vi "Tool Transformation.vi"(2 "SetTRF":sgl[](array[numeric])=[80.67, 0.8359, 79.37, 0.0, 0.0, 0.0] step=1 format="%.3f", 3 "External force":T1 {"£nez" format="%.3f"; "£ney" format="%.3f"; "£nex" format="%.3f"; "Fez" format="%.2f"; "Fey" format="%.2f"; "Fex" format="%.2f"}) -> (0 "Rotation Matrix":dbl[][](array[numeric]), 1 "External force":T1 {"£nez" format="%.3f"; "£ney" format="%.3f"; "£nex" format="%.3f"; "Fez" format="%.2f"; "Fey" format="%.2f"; "Fex" format="%.2f"})   [LabVIEW 2018]
uses:
  <vilib>/Analysis/coordinate.llb/Euler Rotation Order.ctl
  <vilib>/Analysis/Matrix/Datatypes/RealMatrix.ctl
  <vilib>/Analysis/baseanly.llb/A x Vector.vi
  <vilib>/Analysis/baseanly.llb/Real A x B.vi
  <vilib>/Analysis/7linalg.llb/Create Special Real Matrix.vi
  <vilib>/Analysis/NI_AALPro.lvlib
  <vilib>/Analysis/Matrix/NI_Matrix.lvlib
  <vilib>/Analysis/NI_AALBase.lvlib
panel:
  out "Force Check":dbl[](array[numeric])
  out "Torque Check":dbl[](array[numeric])
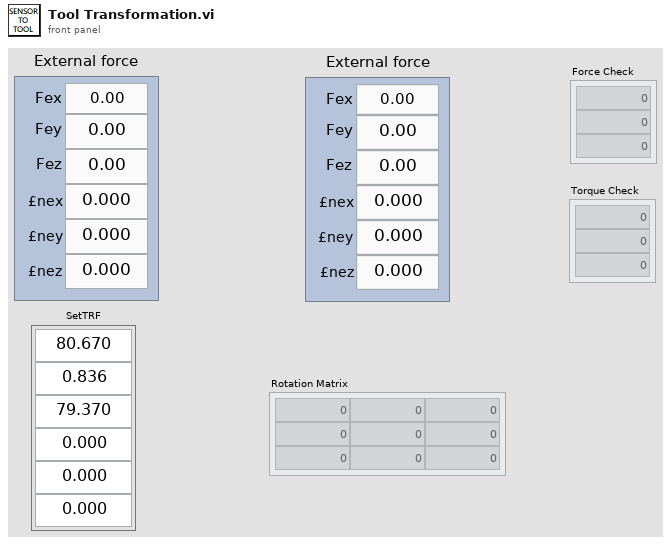
[diagram p1: front panel]
types:
  T1 = cluster{"Fex":dbl, "Fey":dbl, "Fez":dbl, " £nex":dbl, " £ney":dbl, " £nez":dbl}
  T2 = typedef "NI_Matrix.lvlib/RealMatrix.ctl" = dbl[][]
  T3 = typedef "NI_AALPro.lvlib/Euler Rotation Order.ctl" = u16
  T4 = cluster{"Move-SubIndex 1 ":sgl, "Move-SubIndex 1 ":sgl, sgl}
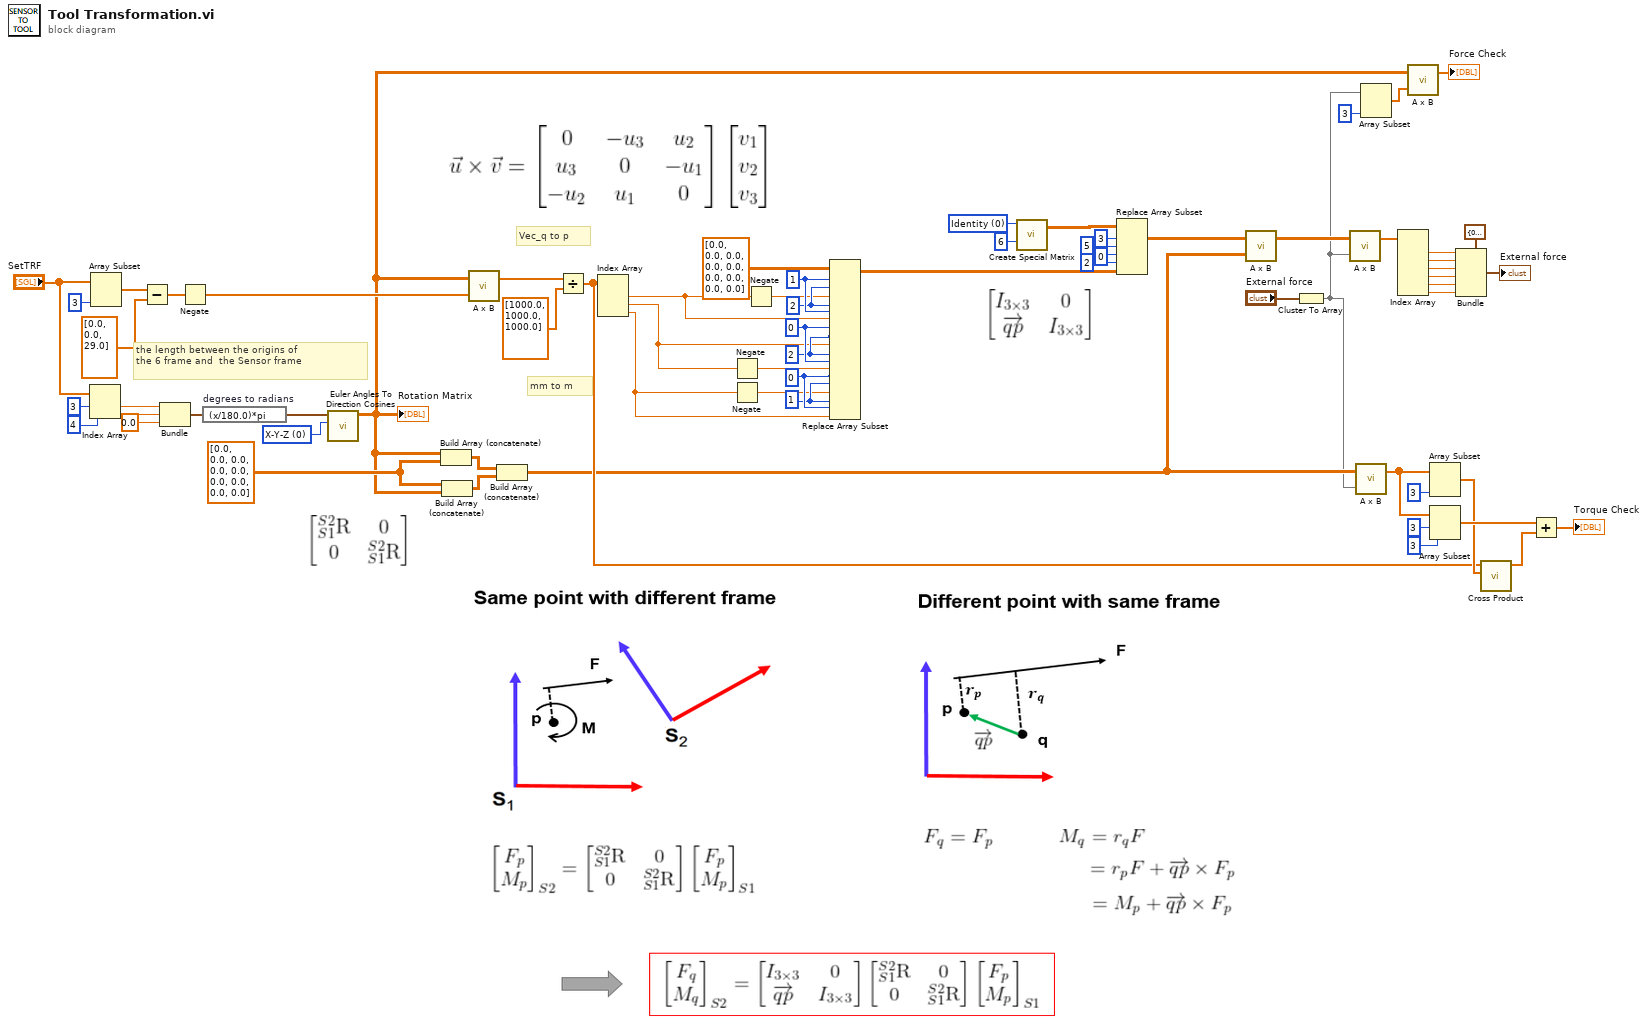
[diagram p0: block diagram]
diagram:
  w40 = T2 [[0.0, 0.0, 0.0], [0.0, 0.0, 0.0], [0.0, 0.0, 0.0]] ("matrix")
  w49 = 1 ("disabled index (col)")
  w50 = 0 ("disabled index (row)")
  w51 = 2 ("disabled index (col)")
  w52 = 0 ("disabled index (row)")
  w53 = 2 ("disabled index (col)")
  w54 = 1 ("disabled index (row)")
  w57 = 0 items=["Identity", "Diagonal", "Toeplitz", "Vandermonde", "Companion", "Hankel", "Hadamard", "Wilkinson", "Hilbert", "Inverse Hilbert", "Rosser", "Pascal"] ("matrix type")
  w66 = T3 0 items=["X-Y-Z", "X-Z-Y", "Y-X-Z", "Y-Z-X", "Z-X-Y", "Z-Y-X", "X-Y-X", "X-Z-X", "Y-X-Y", "Y-Z-Y", "Z-X-Z", "Z-Y-Z"] ("rotation order")
  # "mm to m"
  # "Vec_q to p"
  # "the length between the origins of \nthe 6 frame and  the Sensor frame"
  n1 = Index Array(array="SetTRF", index #1=3 ("index"), index #2=4 ("index")) -> (element #1=w59:sgl, element #2=w58:sgl)
  n2 = Array Subset(array="SetTRF", length=3) -> (w64:sgl[])  [unwired: 1 in]
  n3 = Subtract(x=w64, y=sgl[] [0.0, 0.0, 29.0]) -> (x-y=w12:sgl[])
  n4 = Bundle("Move-SubIndex 1"=w59, "Move-SubIndex 1"=w58, sgl 0.0) -> (w29:T4)  [unwired: 1 in]
  n5 = Negate(x=w12) -> (-x=w9:sgl[])
  n6 = expression code="(x/180.0)*pi" "degrees to radians"(w29) -> (w28:T4)
  n7 = call <vilib>:"Euler Angles To Direction Cosines.vi"("rotation order"=w66, "Euler Angles"=w28) -> ("Direction Cosines"=w1:dbl[][])  [unwired: 8 in, 1 out]
  "Rotation Matrix" <- w1
  n8 = Build Array (concatenate)(w1, w40) -> (w42:T2)
  n9 = Build Array (concatenate)(w40, w1) -> (w41:T2)
  n10 = call-poly <vilib>:"A x B.vi"("Vector"=w9, "A"=w1) -> ("A x Vector"=w8:dbl[])  [unwired: 1 out]
  n11 = Build Array (concatenate)(w42, w41) -> (w7:T2)
  n12 = Divide(x=w8, y=sgl[] [1000.0, 1000.0, 1000.0]) -> (x/y=w11:dbl[])
  n13 = Index Array(array=w11) -> (element #1=w25:dbl, element #2=w26:dbl, element #3=w22:dbl)  [unwired: 3 in]
  n14 = Negate(x=w26) -> (-x=w24:dbl)
  n15 = Negate(x=w22) -> (-x=w23:dbl)
  n16 = Negate(x=w25) -> (-x=w27:dbl)
  n17 = Replace Array Subset(array=T2 [[0.0, 0.0, 0.0], [0.0, 0.0, 0.0], [0.0, 0.0, 0.0]] ("matrix"), new element #1=w27, index (row) #1=w54, index (col) #1=w53, new element #2=w25, index (row) #2=w53, index (col) #2=w54, new element #3=w26, index (row) #3=w52, index (col) #3=w51, new element #4=w24, index (row) #4=w51, index (col) #4=w52, new element #5=w23, index (row) #5=w50, index (col) #5=w49, new element #6=w22, index (row) #6=w49, index (col) #6=w50) -> (w48:T2)
  n18 = call-poly <vilib>:"Create Special Matrix.vi"("matrix type"=w57, "matrix size"=6) -> ("Special Matrix"=w55:T2)  [unwired: 3 in, 1 out]
  n19 = Replace Array Subset(array=w55, new element=w48, index (dim 0)=3 ("row 1"), index (dim 1)=5 ("row N"), index (dim 2)=0 ("row N"), index (dim 3)=2 ("column N")) -> (w6:T2)
  n20 = call-poly <vilib>:"A x B.vi"("B"=w7, "A"=w6) -> ("A x B"=w13:T2)  [unwired: 1 out]
  n21 = Cluster To Array(cluster="External force") -> (array=w4:dbl[])
  n22 = call-poly <vilib>:"A x B.vi"("Vector"=w4, "A"=w13) -> ("A x Vector"=w36:dbl[])  [unwired: 1 out]
  n23 = call-poly <vilib>:"A x B.vi"("Vector"=w4, "A"=w7) -> ("A x Vector"=w14:dbl[])  [unwired: 1 out]
  n24 = Array Subset(array=w4, length=3) -> (w3:dbl[])  [unwired: 1 in]
  n25 = Index Array(array=w36) -> (element #1=w35:dbl, element #2=w34:dbl, element #3=w33:dbl, element #4=w32:dbl, element #5=w31:dbl, element #6=w30:dbl)  [unwired: 6 in]
  n26 = call-poly <vilib>:"A x B.vi"("Vector"=w3, "A"=w1) -> ("A x Vector"=→"Force Check":dbl[])  [unwired: 1 out]
  n27 = Array Subset(array=w14, length=3) -> (w17:dbl[])  [unwired: 1 in]
  n28 = Array Subset(array=w14, index=3, length=3) -> (w18:dbl[])
  n29 = Bundle(cluster=T1 {"Fex"=0.0, "Fey"=0.0, "Fez"=0.0, " £nex"=0.0, " £ney"=0.0, " £nez"=0.0} ("External force"), "Fex"=w35, "Fey"=w34, "Fez"=w33, "£nex"=w32, "£ney"=w31, "£nez"=w30) -> (→"External force":T1)
  n30 = call <vilib>:"Cross Product.vi"("B Vector"=w17, "A Vector"=w11) -> ("Cross Product"=w16:dbl[])  [unwired: 8 in, 1 out]
  n31 = Add(x=w18, y=w16) -> (x+y=→"Torque Check":dbl[])
